vi "Execute.vi"(8 "error in (no error)":errorcluster, 9 "Workspace":T1, 10 "Control In":T2={"I-O.lvclass"=refnum, "Motion.lvclass"=refnum, "Dispenser.lvclass"=refnum}, 11 "Pick and Place in":refnum<class "Pick and Place.lvclass">) -> (0 "error out":errorcluster, 2 "Control Out":T2, 3 "Pick and Place out":refnum<class "Pick and Place.lvclass">)   [LabVIEW 2016, in "Pick and Place.lvclass"]
uses:
  Pick and Place.lvclass
  Controller/Controllers.ctl
  Controller/I-O/I-O.lvclass
  Controller/Motion/A3200/A3200.lvclass
  Controller/Dispenser/Dispenser.lvclass
  Controller/Motion/Motion.lvclass
  Workspace/Workspace.ctl
  Pick and Place.lvclass/Pick and Place.ctl
  Controller/Controller.lvclass
  Workspace/Fixture.lvclass
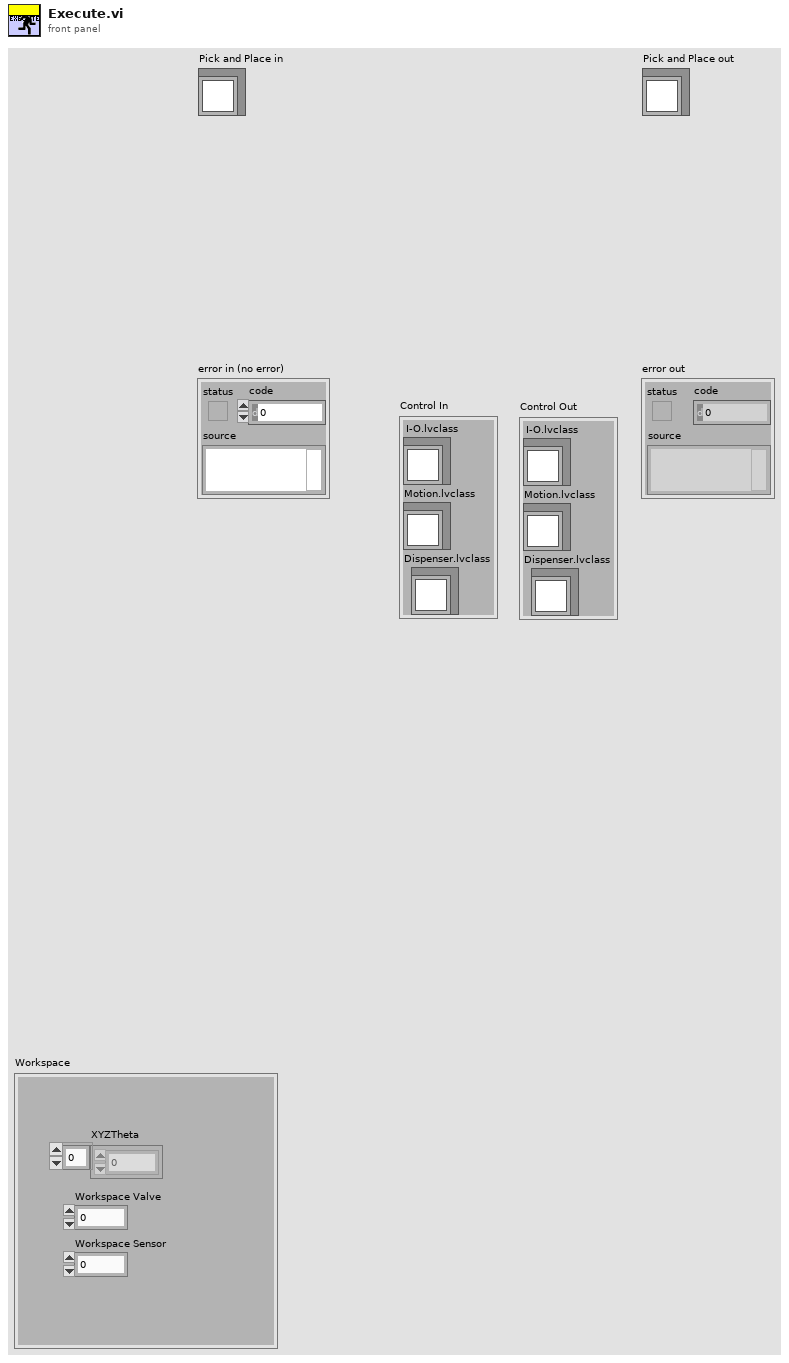
[diagram p1: front panel]
types:
  T1 = typedef "Fixture.lvclass/Workspace.ctl" = cluster{"XYZTheta":dbl[], "Workspace Valve":i32, "Workspace Sensor":i32}
  T2 = typedef "Controller.lvclass/Controllers.ctl" = cluster{"I-O.lvclass":refnum<class "I-O.lvclass">, "Motion.lvclass":refnum<class "Motion.lvclass">, "Dispenser.lvclass":refnum<class "Dispenser.lvclass">}
  T3 = typedef "Pick and Place.lvclass/Pick and Place Type.ctl" = enum16{"Primary Pick Up", "Secondary Pick Up", "Put Down All", "Pick Up All", "Put Down Secondary"}
  T4 = typedef "I-O.lvclass/Pin Map.ctl" = cluster{"Region Valves":i32[], "Extra Valves":dbl[][][], "Tool Primary Valve":i32, "Tool Secondary Valve":i32, "Region Sensors":i32[], "Extra Sensors":dbl[][][], "Tool Primary Sensor":dbl, "Tool Secondary Sensor":dbl, "Compression Sensor":dbl, "5V":i32}
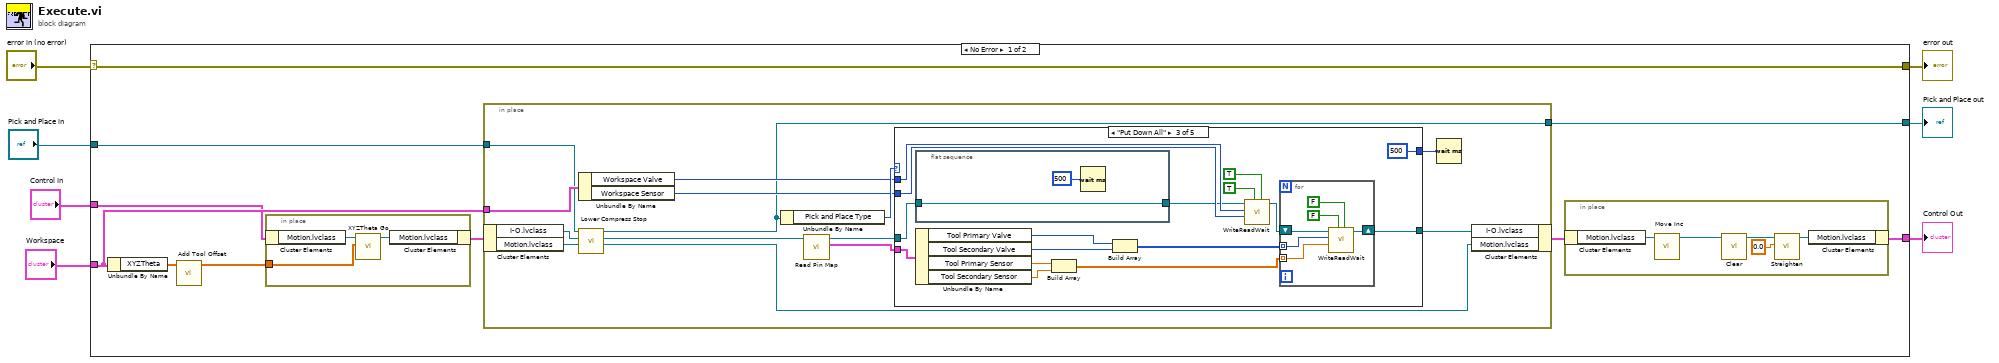
[diagram p0: block diagram]
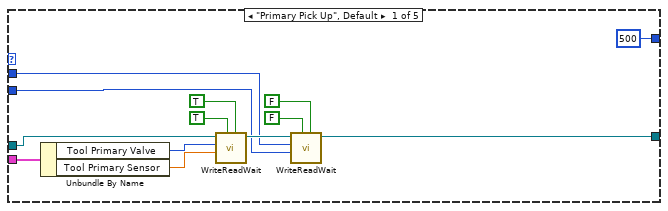
[diagram p2: hidden frame]
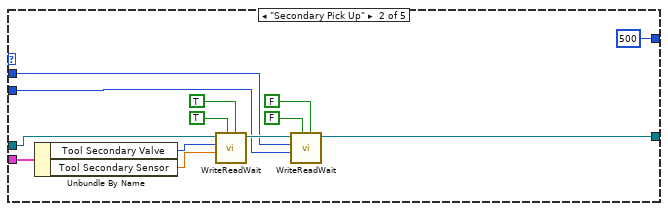
[diagram p3: hidden frame]
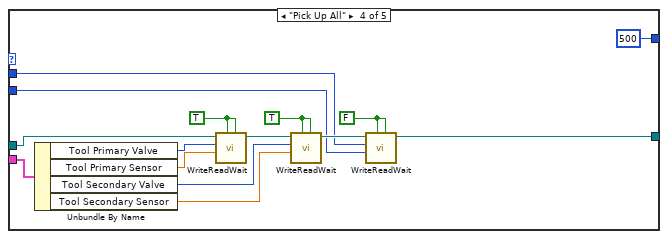
[diagram p4: hidden frame]
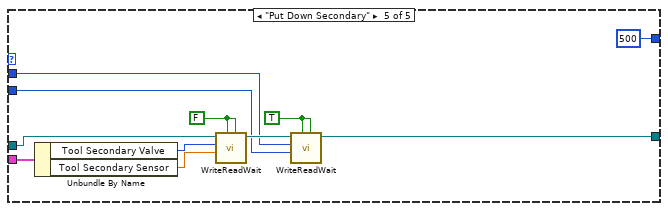
[diagram p5: hidden frame]
diagram:
  n1 = case shown="No Error" "error in (no error)" {
    selector: "error in (no error)" -> [w17 w117]
    tunnel: "Control In" -> [w13 w118]
    tunnel: "Workspace" -> [w14 _]
    tunnel: [w17 w117] -> w1
    tunnel: [w12 w118] -> w2
    tunnel: "Pick and Place in" -> [w11 w116]
    tunnel: [w10 w116] -> w6
    frame No Error {
      n2 = Unbundle By Name(w14) -> ("XYZTheta"=w9:dbl[])
      n3 = call "Add Tool Offset.vi"("XYZTheta"=w9) -> ("Array"=w8:dbl[])  [unwired: 10 in]
      n4 = in-place {
        in-place-border: w8 -> [w115]
        n5 = in-place-cluster #1(w13) -> ("Motion.lvclass"=w114:refnum<class "Motion.lvclass">)
        n6 = call "XYZTheta Go.vi"("XYZTheta In"=w115, "Motion in"=w114) -> ("Motion out"=w113:refnum<class "Motion.lvclass">)  [unwired: 7 in, 2 out]
        n7 = in-place-cluster #1("Motion.lvclass"=w113) -> (w16:T2)
      }
      n8 = in-place {
        in-place-border: w14 -> [w31]
        in-place-border: w11 -> [w19]
        in-place-border: [w18] -> w10
        n9 = in-place-cluster #2(w16) -> ("I-O.lvclass"=w24:refnum<class "I-O.lvclass">, "Motion.lvclass"=w23:refnum<class "Motion.lvclass">)
        n10 = Unbundle By Name(w31) -> ("Workspace Valve"=w29:i32, "Workspace Sensor"=w28:i32)
        n11 = call "Lower Compress Stop.vi"("Motion.lvclass"=w23, "I-O.lvclass"=w24, "Pick and Place in"=w19) -> ("Motion.lvclass"=w21:refnum<class "Motion.lvclass">, "I-O out"=w20:refnum<class "I-O.lvclass">, "Pick and Place Out"=w18:refnum<class "Pick and Place.lvclass">)  [unwired: 5 in, 1 out]
        n12 = Unbundle By Name(w18) -> ("Pick and Place Type"=w30:T3)
        n13 = call-dynamic "Read Pin Map.vi"("I-O in"=w20) -> ("Pin Map"=w26:T4, "I-O out"=w25:refnum<class "I-O.lvclass">)  [unwired: 8 in, 1 out]
        n14 = case shown="\"Put Down All\"" w30 {
          tunnel: w29 -> [w41 w49 w63 w86 w101]
          tunnel: w28 -> [w40 w48 w62 w85 w100]
          tunnel: [w35 w47 w67 w83 w98] -> w22
          tunnel: [u32 500 ("milliseconds to wait") 500 500 u32 500 ("milliseconds to wait") u32 500 ("milliseconds to wait")] -> w27
          tunnel: w25 -> [w34 w46 w58 w95 w106]
          tunnel: w26 -> [w33 w45 w61 w96 w107]
          frame "Primary Pick Up", Default {
            n15 = Unbundle By Name(w33) -> ("Tool Primary Valve"=w32:i32, "Tool Primary Sensor"=w43:dbl)
            n16 = call "WriteReadWait.vi"("Read Value"=TRUE, "Write Value"=TRUE, "Read"=w43, "Write"=w32, "I-O in"=w34) -> ("I-O out"=w42:refnum<class "I-O.lvclass">)  [unwired: 5 in, 1 out]
            n17 = call "WriteReadWait.vi"("Read Value"=FALSE ("Write Value"), "Write Value"=FALSE ("Read Value"), "Read"=w40, "Write"=w41, "I-O in"=w42) -> ("I-O out"=w35:refnum<class "I-O.lvclass">)  [unwired: 5 in, 1 out]
          }
          frame "Secondary Pick Up" {
            n18 = Unbundle By Name(w45) -> ("Tool Secondary Valve"=w51:i32, "Tool Secondary Sensor"=w50:dbl)
            n19 = call "WriteReadWait.vi"("Read Value"=TRUE, "Write Value"=TRUE, "Read"=w50, "Write"=w51, "I-O in"=w46) -> ("I-O out"=w56:refnum<class "I-O.lvclass">)  [unwired: 5 in, 1 out]
            n20 = call "WriteReadWait.vi"("Read Value"=FALSE ("Write Value"), "Write Value"=FALSE ("Read Value"), "Read"=w48, "Write"=w49, "I-O in"=w56) -> ("I-O out"=w47:refnum<class "I-O.lvclass">)  [unwired: 5 in, 1 out]
          }
          frame "Put Down All" {
            n21 = flat-sequence {
              tunnel: [w74] -> w59
              tunnel: w58 -> [w74]
              frame #0 {
                # "Delay After Placing"
                n22 = Wait (ms)(milliseconds to wait=u32 500) -> ()  [unwired: 1 out]
              }
            }
            n23 = Unbundle By Name(w61) -> ("Tool Primary Valve"=w68:i32, "Tool Secondary Valve"=w69:i32, "Tool Primary Sensor"=w70:dbl, "Tool Secondary Sensor"=w71:dbl)
            n24 = Build Array(w70, w71) -> (w73:dbl[])
            n25 = Build Array(w68, w69) -> (w72:i32[])
            n26 = call "WriteReadWait.vi"("Read Value"=TRUE, "Write Value"=TRUE, "Read"=w62, "Write"=w63, "I-O in"=w59) -> ("I-O out"=w60:refnum<class "I-O.lvclass">)  [unwired: 5 in, 1 out]
            n27 = for {
              shift-right: [w76] -> w67
              shift-left: w60 -> [w77]
              tunnel: w72 -> [w79] mode=indexing
              tunnel: w73 -> [w78] mode=indexing
              n28 = call "WriteReadWait.vi"("Read Value"=FALSE ("Write Value"), "Write Value"=FALSE ("Read Value"), "Read"=w78, "Write"=w79, "I-O in"=w77) -> ("I-O out"=w76:refnum<class "I-O.lvclass">)  [unwired: 5 in, 1 out]
            }
          }
          frame "Pick Up All" {
            w84 = FALSE ("Read Value")
            w88 = TRUE ("Write Value")
            w94 = TRUE ("Write Value")
            n29 = Unbundle By Name(w96) -> ("Tool Primary Valve"=w93:i32, "Tool Primary Sensor"=w92:dbl, "Tool Secondary Valve"=w90:i32, "Tool Secondary Sensor"=w89:dbl)
            n30 = call "WriteReadWait.vi"("Read Value"=w94, "Write Value"=w94, "Read"=w92, "Write"=w93, "I-O in"=w95) -> ("I-O out"=w91:refnum<class "I-O.lvclass">)  [unwired: 5 in, 1 out]
            n31 = call "WriteReadWait.vi"("Read Value"=w88, "Write Value"=w88, "Read"=w89, "Write"=w90, "I-O in"=w91) -> ("I-O out"=w87:refnum<class "I-O.lvclass">)  [unwired: 5 in, 1 out]
            n32 = call "WriteReadWait.vi"("Read Value"=w84, "Write Value"=w84, "Read"=w85, "Write"=w86, "I-O in"=w87) -> ("I-O out"=w83:refnum<class "I-O.lvclass">)  [unwired: 5 in, 1 out]
          }
          frame "Put Down Secondary" {
            w99 = TRUE ("Read Value")
            w103 = FALSE ("Write Value")
            n33 = Unbundle By Name(w107) -> ("Tool Secondary Valve"=w105:i32, "Tool Secondary Sensor"=w104:dbl)
            n34 = call "WriteReadWait.vi"("Read Value"=w103, "Write Value"=w103, "Read"=w104, "Write"=w105, "I-O in"=w106) -> ("I-O out"=w102:refnum<class "I-O.lvclass">)  [unwired: 5 in, 1 out]
            n35 = call "WriteReadWait.vi"("Read Value"=w99, "Write Value"=w99, "Read"=w100, "Write"=w101, "I-O in"=w102) -> ("I-O out"=w98:refnum<class "I-O.lvclass">)  [unwired: 5 in, 1 out]
          }
        }
        n36 = Wait (ms)(milliseconds to wait=w27) -> ()  [unwired: 1 out]
        n37 = in-place-cluster #2("I-O.lvclass"=w22, "Motion.lvclass"=w21) -> (w15:T2)
      }
      n38 = in-place {
        n39 = in-place-cluster #3(w15) -> ("Motion.lvclass"=w108:refnum<class "Motion.lvclass">)
        n40 = call-dynamic "Move Inc.vi"("Motion in"=w108) -> ("Motion out"=w109:refnum<class "Motion.lvclass">)  [unwired: 9 in, 1 out]
        n41 = call "Clear.vi"("Motion in"=w109) -> ("Motion out"=w112:refnum<class "Motion.lvclass">)  [unwired: 9 in, 1 out]
        n42 = call-dynamic "Straighten.vi"("Theta"=0.0 ("Angle (rad)"), "Motion in"=w112) -> ("Motion out"=w111:refnum<class "Motion.lvclass">)  [unwired: 8 in, 1 out]
        n43 = in-place-cluster #3("Motion.lvclass"=w111) -> (w12:T2)
      }
    }
    frame Error {
    }
  }
  "error out" <- w1
  "Pick and Place out" <- w6
  "Control Out" <- w2
